vi "FP Comm Protocol.vi"() -> ()   [LabVIEW 2021]
uses:
  Comm Protocol/Comm Protocol.lvclass
panel:
  in  "Comm Protocol.lvclass":refnum<class "Comm Protocol.lvclass">
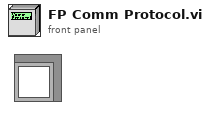
[diagram p1: front panel]
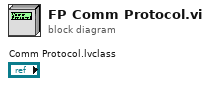
[diagram p0: block diagram]
diagram:
